vi "set_minimum_output_value.vi"(8 "error in (no error)":errorcluster, 10 "minimum output value":dbl, 11 "DAQmxWriteSignals.lvclass in":refnum<class "SignalWriterDL090202DAQmx.lvclass">) -> (0 "error out":errorcluster, 3 "DAQmxWriteSignals.lvclass out":refnum<class "SignalWriterDL090202DAQmx.lvclass">)   [LabVIEW 2010, in "SignalWriterDL090202DAQmx.lvclass"]
uses:
  SignalWriterDL090202DAQmx.lvclass
  GenericSignalWriter/GenericSignalWriter/GenericSignalWriter.lvclass
  SignalWriterDL090202DAQmx.lvclass/SignalWriterDL090202DAQmx.ctl
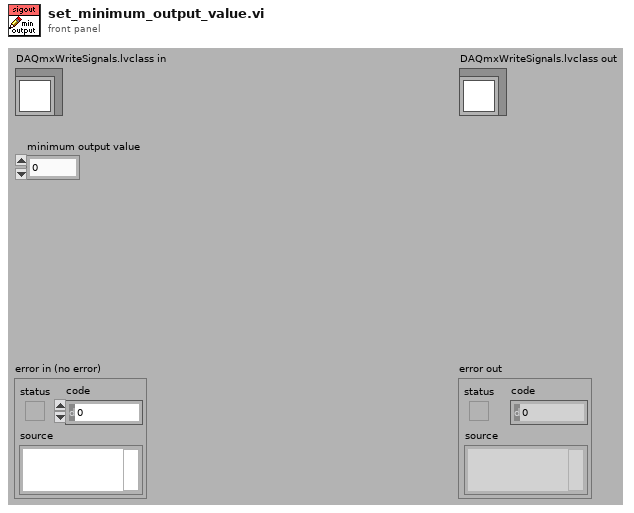
[diagram p1: front panel]
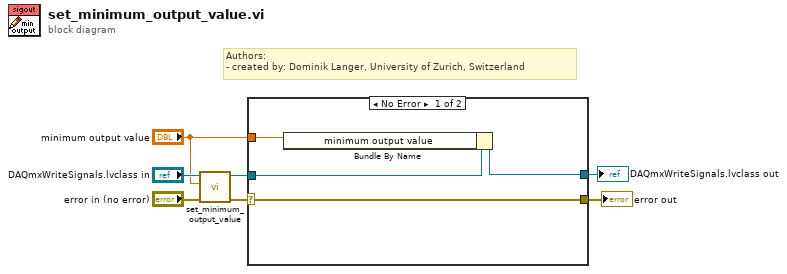
[diagram p0: block diagram]
diagram:
  # "Authors: \n- created by: Dominik Langer, University of Zurich, Switzerland"
  n1 = call-parent "set_minimum_output_value.vi"("error in (no error)"="error in (no error)", "minimum output value"="minimum output value", "GenericWriteSignals.lvclass in"="DAQmxWriteSignals.lvclass in") -> ("error out"=w5:errorcluster, "GenericWriteSignals.lvclass out"=w4:refnum<class "SignalWriterDL090202DAQmx.lvclass">)  [unwired: 7 out]
  n2 = case shown="No Error" w5 {
    selector: w5 -> [w9 w12]
    tunnel: w4 -> [w11 w13]
    tunnel: [w10 w13] -> w3
    tunnel: [w9 w12] -> w2
    tunnel: "minimum output value" -> [w8 _]
    frame No Error {
      n3 = Bundle By Name(cluster=w11, "minimum output value"=w8) -> (w10:refnum<class "SignalWriterDL090202DAQmx.lvclass">)
    }
    frame Error {
    }
  }
  "error out" <- w2
  "DAQmxWriteSignals.lvclass out" <- w3
